vi "oa_TV Check Number of Channels.vi"(0 "missing pulses? (no:F)":bool[](array[boolean]), 1 "threshold (auto)":dbl[](array[numeric]) format="%.2f", 2 "pulse/revolution (1)":i32[](array[numeric]), 3 "hysteresis (0)":dbl[](array[numeric]), 4 "pulse width (2)":i32[](array[numeric]), 5 "error in (no error)":errorcluster, 6 "channel number":i32, 7 "slope (Rising)":u16[](array[ring]) items=["Rising", "Falling"], 10 "tacho selection":enum16{"Analog Tacho", "Digital Tacho"}(ring)) -> (13 "slope out":u16[](array[ring]) items=["Rising", "Falling"], 14 "missing pulses? out":bool[](array[boolean]), 15 "threshold out":dbl[](array[numeric]) format="%.2f", 16 "pulse/revolution out":i32[](array[numeric]), 17 "hysteresis out":dbl[](array[numeric]), 18 "pulse width out":i32[](array[numeric]), 19 "error out":errorcluster)   [LabVIEW 2017, in "SoundVib_Torsional.lvlib"]
uses:
  <vilib>/addons/Sound and Vibration/Order Analysis/Torsional Vibration/SoundVib_Torsional.lvlib
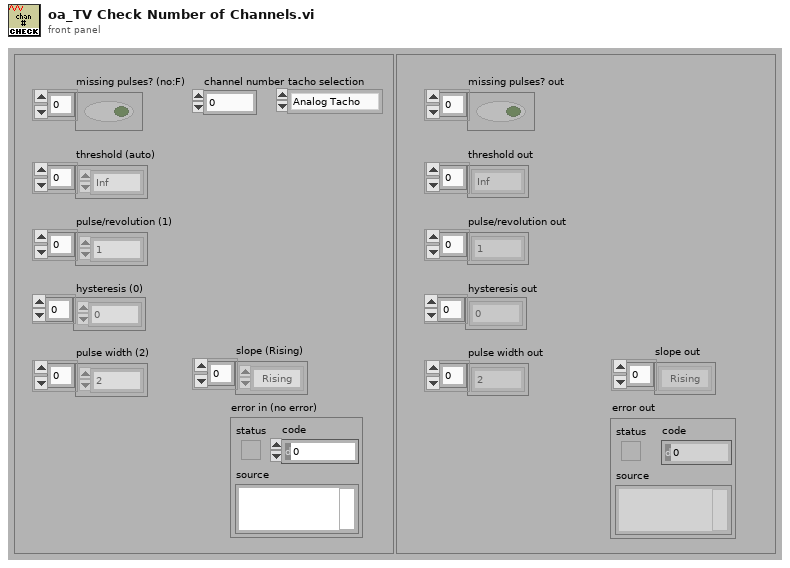
[diagram p1: front panel]
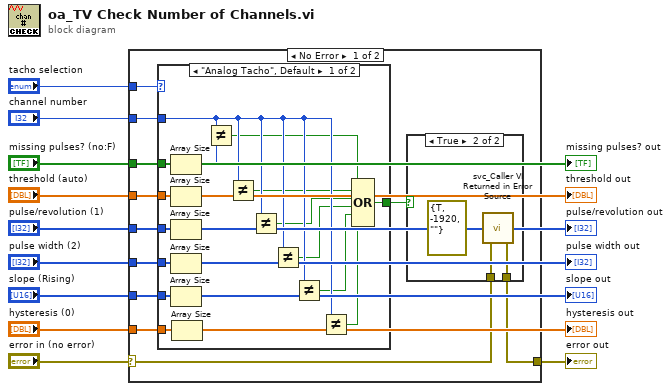
[diagram p0: block diagram]
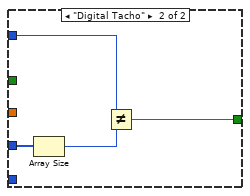
[diagram p2: hidden frame]
diagram:
  n1 = case shown="No Error" "error in (no error)" {
    selector: "error in (no error)" -> [w16 w50]
    tunnel: [w15 w50] -> w9
    tunnel: "missing pulses? (no:F)" -> [w21 _]
    tunnel: "threshold (auto)" -> [w20 _]
    tunnel: "channel number" -> [w13 _]
    tunnel: "pulse/revolution (1)" -> [w19 _]
    tunnel: "pulse width (2)" -> [w18 _]
    tunnel: "slope (Rising)" -> [w17 _]
    tunnel: "hysteresis (0)" -> [w14 _]
    tunnel: "tacho selection" -> [w11 _]
    frame No Error {
      n2 = case shown="\"Analog Tacho\", Default" w11 {
        tunnel: w21 -> [w41 _]
        tunnel: w20 -> [w40 _]
        tunnel: w19 -> [w39 w45]
        tunnel: w18 -> [w38 _]
        tunnel: w17 -> [w37 _]
        tunnel: w14 -> [w36 _]
        tunnel: w13 -> [w35 w44]
        tunnel: [w25 w42] -> w12
        frame "Analog Tacho", Default {
          n3 = Array Size(array=w41) -> (size(s)=w34:i32)
          n4 = Array Size(array=w40) -> (size(s)=w33:i32)
          n5 = Array Size(array=w39) -> (size(s)=w32:i32)
          n6 = Array Size(array=w38) -> (size(s)=w31:i32)
          n7 = Array Size(array=w37) -> (size(s)=w30:i32)
          n8 = Array Size(array=w36) -> (size(s)=w23:i32)
          n9 = Not Equal?(x=w35, y=w34) -> (x != y?=w29:bool)
          n10 = Not Equal?(x=w35, y=w33) -> (x != y?=w28:bool)
          n11 = Not Equal?(x=w35, y=w32) -> (x != y?=w27:bool)
          n12 = Not Equal?(x=w35, y=w31) -> (x != y?=w26:bool)
          n13 = Not Equal?(x=w35, y=w30) -> (x != y?=w24:bool)
          n14 = Not Equal?(x=w35, y=w23) -> (x != y?=w22:bool)
          n15 = Compound Arithmetic op=OR(w29, w28, w27, w26, w24, w22) -> (w25:bool)
        }
        frame "Digital Tacho" {
          n16 = Array Size(array=w45) -> (size(s)=w43:i32)
          n17 = Not Equal?(x=w44, y=w43) -> (x != y?=w42:bool)
        }
      }
      n18 = case shown="True" w12 {
        tunnel: w16 -> [w46 w48]
        tunnel: [w46 w47] -> w15
        frame False {
        }
        frame True {
          n19 = call <vilib>:"svc_Caller VI Returned in Error Source.vi"("warning input to caller"=w48, "error in (no error)"=errorcluster {"status"=TRUE, "code"=-1920, "source"=""} ("error out")) -> ("error out"=w47:errorcluster)  [unwired: 3 in]
        }
      }
    }
    frame Error {
    }
  }
  "error out" <- w9
  "threshold out" <- "threshold (auto)"
  "pulse/revolution out" <- "pulse/revolution (1)"
  "pulse width out" <- "pulse width (2)"
  "slope out" <- "slope (Rising)"
  "missing pulses? out" <- "missing pulses? (no:F)"
  "hysteresis out" <- "hysteresis (0)"
